vi "timing and stabilization test.vi"() -> ()   [LabVIEW 2013]
uses:
  MeasurementControl Message Queue Folder/MeasurementControl Message Queue.lvlib
panel:
  in  "Start Insulated Sphere Timer":bool
  in  "Reset Insulated Sphere Timer":bool
  in  "Start Naked Sphere Timer":bool
  out "Message":string
  in  "Reset Naked Sphere Timer":bool
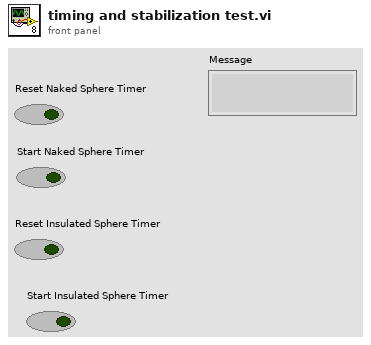
[diagram p1: front panel]
types:
  T1 = typedef "MeasurementControl Message Queue.lvlib/All Message Queues.ctl" = cluster{"Master":refnum<queue>, "UI":refnum<queue>, "Stabilization":refnum<queue>, "Logging":refnum<queue>, "Timing":refnum<queue>}
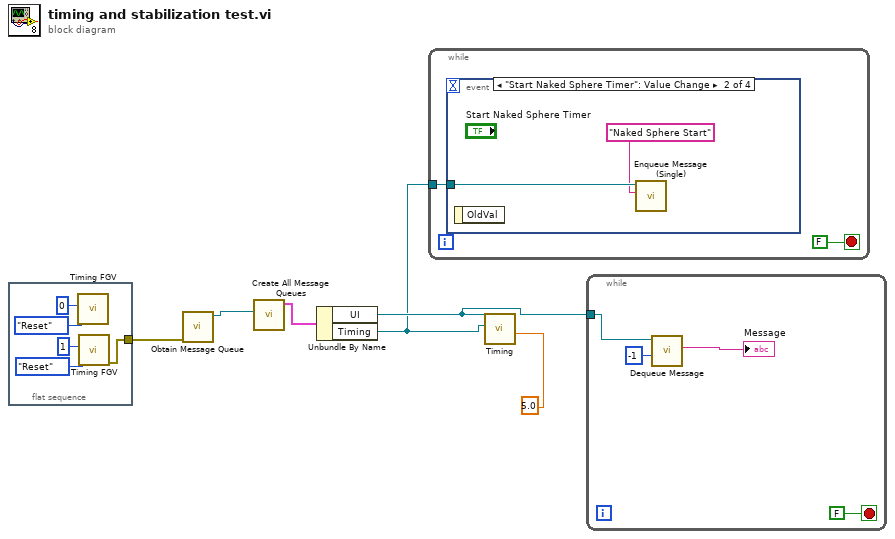
[diagram p0: block diagram]
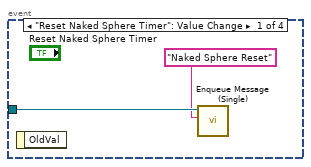
[diagram p2: hidden frame]
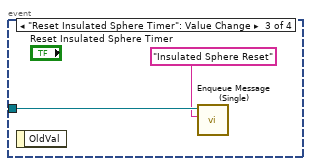
[diagram p3: hidden frame]
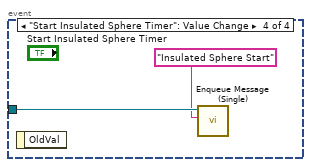
[diagram p4: hidden frame]
diagram:
  n1 = flat-sequence {
    tunnel: [w7] -> w1
    frame #0 {
      n2 = call "Timing FGV.vi"("Index"=0, "Method (Get Time)"=enum16{"Start", "Stop", "Reset", "Get Time"}."Reset") -> ()  [unwired: 7 in, 3 out]
      n3 = call "Timing FGV.vi"("Index"=1, "Method (Get Time)"=enum16{"Start", "Stop", "Reset", "Get Time"}."Reset") -> ("error out"=w7:errorcluster)  [unwired: 7 in, 2 out]
    }
  }
  n4 = call "Obtain Message Queue.vi"("error in (no error)"=w1) -> ("Message Queue"=w6:refnum<queue>)  [unwired: 9 in, 1 out]
  n5 = call "Create All Message Queues.vi"("Master Queue In"=w6) -> ("Message Queues out"=w5:T1)  [unwired: 9 in, 1 out]
  n6 = Unbundle By Name(w5) -> ("UI"=w3:refnum<queue>, "Timing"=w2:refnum<queue>)
  n7 = while {
    tunnel: w2 -> [w13]
    stop <- FALSE stop-if-true
    n8 = event shown="[1] \"Start Naked Sphere Timer\": Value Change" {
      selector: _ -> [_ _ _ _]
      dyn-events: _ -> [_ _ _ _]
      timeout: _ -> [_ _ _ _]
      tunnel: w13 -> [w15 w17 w19 w21]
      event "Reset Naked Sphere Timer": Value Change {
        n9 = event-data() -> ()  [unwired: 1 in, 1 out]
        n10 = call "Enqueue Message (Single).vi"("Message"="Naked Sphere Reset", "Message Queue"=w15) -> ()  [unwired: 8 in, 2 out]
      }
      event "Start Naked Sphere Timer": Value Change {
        n11 = event-data() -> ()  [unwired: 1 in, 1 out]
        n12 = call "Enqueue Message (Single).vi"("Message"="Naked Sphere Start", "Message Queue"=w17) -> ()  [unwired: 8 in, 2 out]
      }
      event "Reset Insulated Sphere Timer": Value Change {
        n13 = event-data() -> ()  [unwired: 1 in, 1 out]
        n14 = call "Enqueue Message (Single).vi"("Message"="Insulated Sphere Reset", "Message Queue"=w19) -> ()  [unwired: 8 in, 2 out]
      }
      event "Start Insulated Sphere Timer": Value Change {
        n15 = event-data() -> ()  [unwired: 1 in, 1 out]
        n16 = call "Enqueue Message (Single).vi"("Message"="Insulated Sphere Start", "Message Queue"=w21) -> ()  [unwired: 8 in, 2 out]
      }
    }
  }
  n17 = call "Timing.vi"("Stabilization\nInterval"=5.0 ("Stabilization\nInterval"), "Timing"=w2, "UI"=w3) -> ()  [unwired: 8 in, 1 out]
  n18 = while {
    tunnel: w3 -> [w25]
    stop <- FALSE stop-if-true
    n19 = call "Dequeue Message.vi"("timeout in ms (-1)"=-1, "Message Queue"=w25) -> ("Message"=→"Message":string)  [unwired: 6 in, 3 out]
  }
